vi "_Main.vi"   [LabVIEW 2017, in "Compressor.lvlib"]
uses:
  Compressor.lvlib
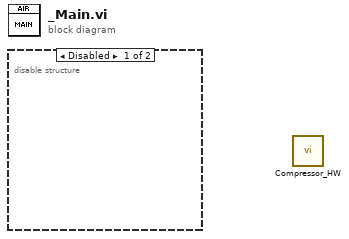
[diagram p0: block diagram]
diagram:
  n1 = disable-structure shown="Disabled" {
    frame Disabled {
    }
    frame Enabled {
    }
  }
  n2 = call "Compressor_HW.vi"() -> ()  [unwired: 12 in]
